vi "CAN Tx Q Ref Init.vi"(6 "CAN FGV State":T1=enum."Get", 8 "error in":errorcluster, 10 "Current Scoket":i16, 11 "queue in":refnum<queue>) -> (0 "error out":errorcluster, 3 "CAN TX queue out":refnum<queue>)   [LabVIEW 2023, in "LTT_TeststandSteptypes.lvlib"]
uses:
  LTT_TeststandSteptypes.lvlib
  Control/CAN FGV State.ctl
  <vilib>/xnet/xnet.llb/XNET Frame CAN.ctl
  <vilib>/xnet/xnet.llb/XNET Frame Type CAN.ctl
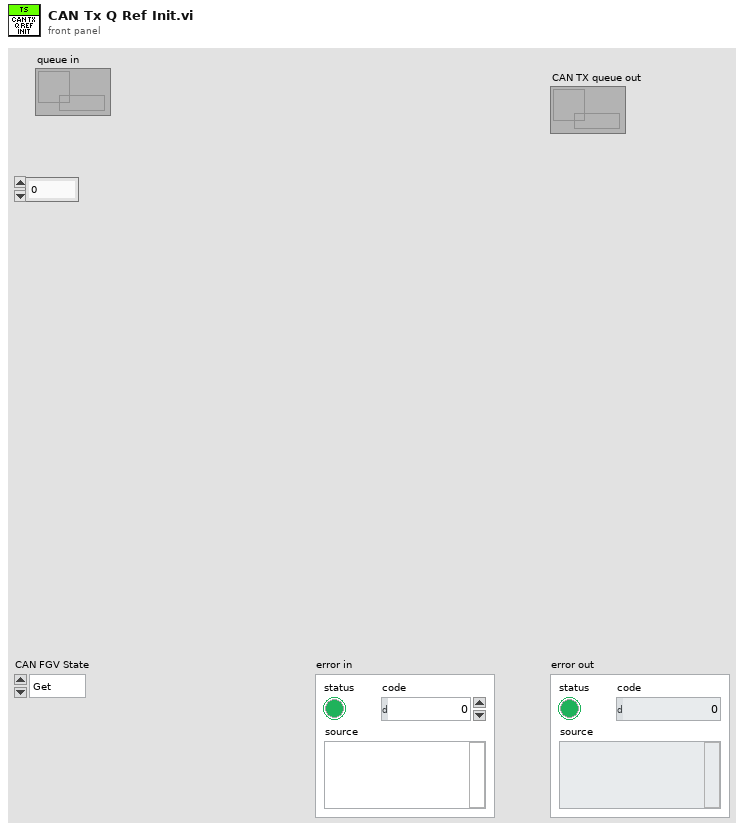
[diagram p1: front panel]
types:
  T1 = typedef "LTT_TeststandSteptypes.lvlib/CAN FGV State.ctl" = enum16{"Init", "Get", "Set"}
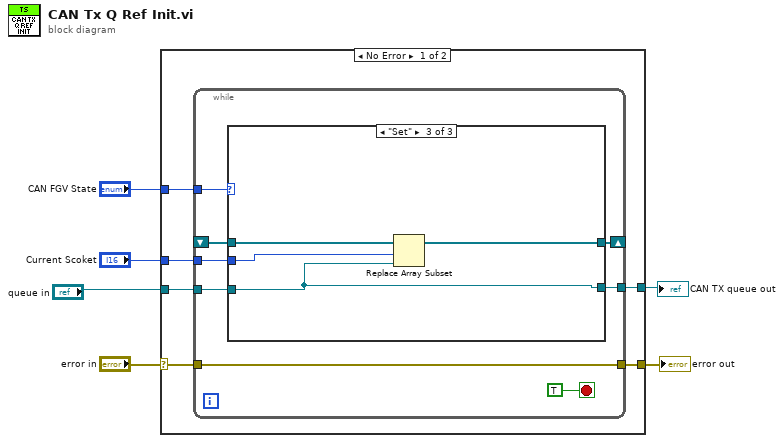
[diagram p0: block diagram]
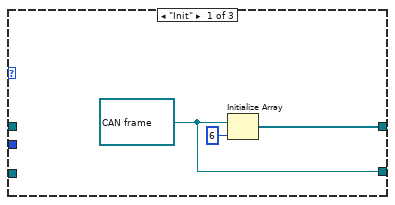
[diagram p2: hidden frame]
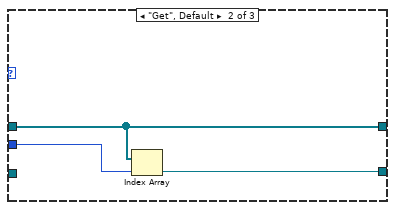
[diagram p3: hidden frame]
diagram:
  n1 = case shown="No Error" "error in" {
    selector: "error in" -> [w12 w31]
    tunnel: "CAN FGV State" -> [w11 _]
    tunnel: [w10 w31] -> w4
    tunnel: "queue in" -> [w9 _]
    tunnel: "Current Scoket" -> [w8 _]
    tunnel: [w7 _] -> w1
    frame No Error {
      n2 = while {
        tunnel: w12 -> [w16]
        tunnel: w11 -> [w19]
        shift-right: [w18] -> _
        shift-left: _ -> [w17]
        tunnel: [w16] -> w10
        tunnel: w9 -> [w15]
        tunnel: w8 -> [w14]
        tunnel: [w13] -> w7
        stop <- TRUE stop-if-true
        n3 = case shown="\"Set\"" w19 {
          tunnel: [w22 w26 w29] -> w18
          tunnel: w17 -> [_ w26 w30]
          tunnel: w15 -> [_ _ w27]
          tunnel: w14 -> [_ w25 w28]
          tunnel: [w21 w24 w27] -> w13
          frame "Init" {
            w21 = refnum<queue> refnum ("queue in")
            n4 = Initialize Array(w21, 6 ("dimension size")) -> (w22:refnum<queue>[])
          }
          frame "Get", Default {
            n5 = Index Array(array=w26, index=w25) -> (element=w24:refnum<queue>)
          }
          frame "Set" {
            n6 = Replace Array Subset(array=w30, new element=w27, index=w28) -> (w29:refnum<queue>[])
          }
        }
      }
    }
    frame Error {
    }
  }
  "error out" <- w4
  "CAN TX queue out" <- w1
